vi "BoxCarAverager.vi"(10 "Bin Size":i32, 11 "Graph in":cluster{dbl[], dbl[]}) -> (1 "SE":dbl[](array[numeric]), 2 "SD":dbl[](array[numeric]), 3 "Graph out":cluster{dbl[], dbl[]})   [LabVIEW 2019]
uses:
  <vilib>/Analysis/NI_AALBase.lvlib
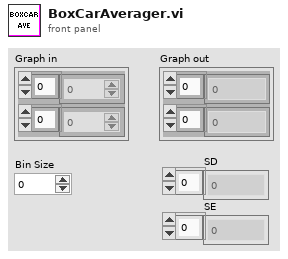
[diagram p1: front panel]
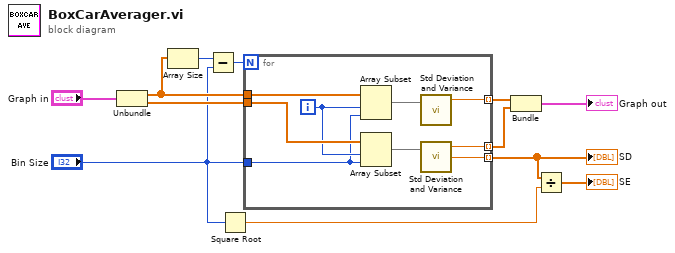
[diagram p0: block diagram]
diagram:
  n1 = Unbundle("Graph in") -> (w11:dbl[], w12:dbl[])
  n2 = Array Size(array=w11) -> (size(s)=w7:i32)
  n3 = Subtract(x=w7, y="Bin Size") -> (x-y=w5:i32)
  n4 = Square Root(x="Bin Size") -> (sqrt(x)=w2:dbl)
  n5 = for {
    N: w5 -> [_]
    tunnel: w11 -> [w18]
    tunnel: w12 -> [w21]
    tunnel: "Bin Size" -> [w19]
    tunnel: [w15] -> w9 mode=indexing
    tunnel: [w14] -> w6 mode=indexing
    tunnel: [w13] -> w4 mode=indexing
    i -> [w20]
    n6 = Array Subset(array=w18, index=w20, length=w19) -> (w17:dbl[])
    n7 = Array Subset(array=w21, index=w20, length=w19) -> (w16:dbl[])
    n8 = call <vilib>:"Std Deviation and Variance.vi"("X"=w17) -> ("mean"=w15:dbl)  [unwired: 1 in, 2 out]
    n9 = call <vilib>:"Std Deviation and Variance.vi"("X"=w16) -> ("mean"=w14:dbl, "standard deviation"=w13:dbl)  [unwired: 1 in, 1 out]
  }
  "SD" <- w4
  n10 = Bundle(w9, w6) -> (→"Graph out":cluster{dbl[], dbl[]})  [unwired: 1 in]
  n11 = Divide(x=w4, y=w2) -> (x/y=→"SE":dbl[])
